vi "photometric acquisitions.vi"(8 "error in (no error)":errorcluster, 11 "S4GEI in":refnum<class "S4GEI.lvclass">) -> (0 "error out":errorcluster, 3 "S4GEI out":refnum<class "S4GEI.lvclass">)   [LabVIEW 2018, in "S4GEI.lvclass"]
uses:
  S4GEI.lvclass
  S4GEI.lvclass/S4GEI.ctl
  State Machine/State Machine.lvclass
  Channel GUI/Channel.lvclass
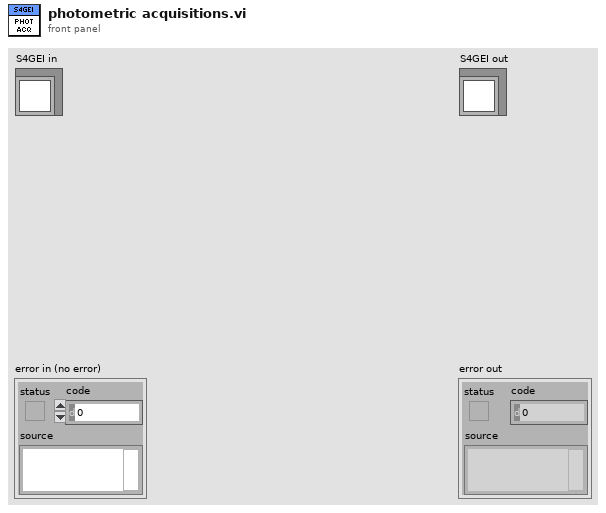
[diagram p1: front panel]
types:
  T1 = cluster{"Acquire":bool, "Stop Acquisition":bool, "Abort Acquisition":bool, "Pause acquisition":bool}
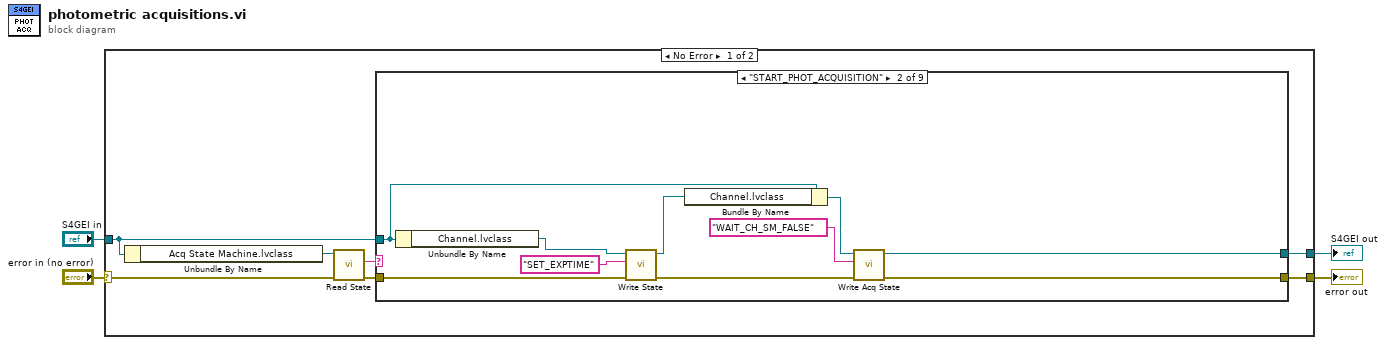
[diagram p0: block diagram]
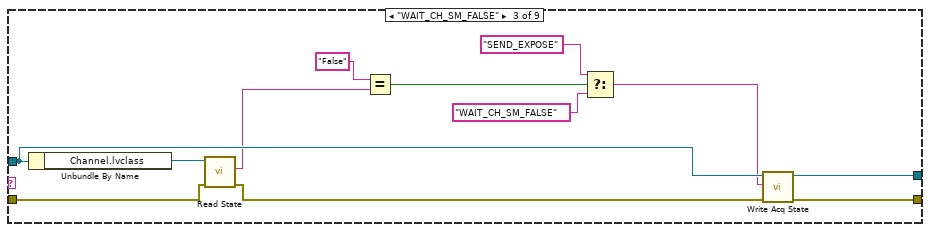
[diagram p3: hidden frame]
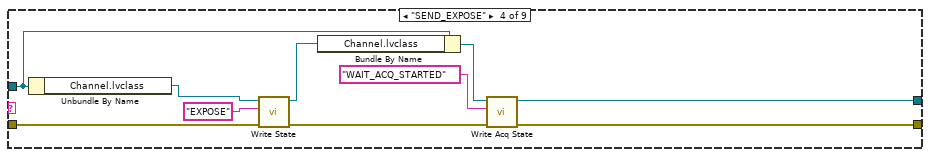
[diagram p4: hidden frame]
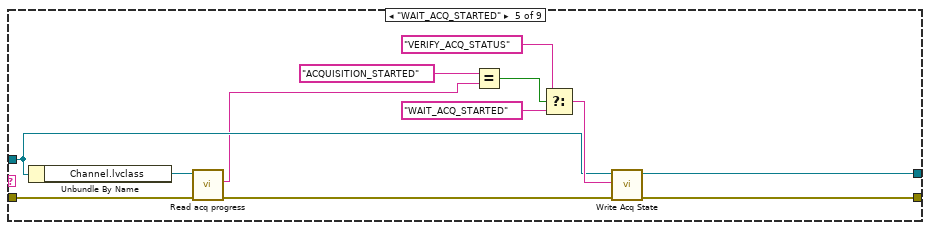
[diagram p5: hidden frame]
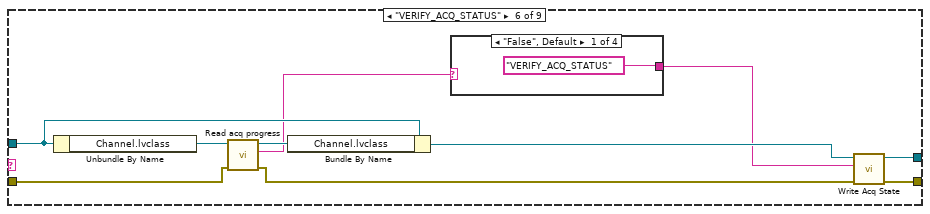
[diagram p6: hidden frame]
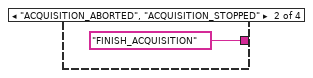
[diagram p7: hidden frame]
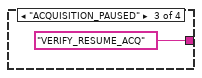
[diagram p8: hidden frame]
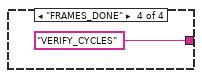
[diagram p9: hidden frame]
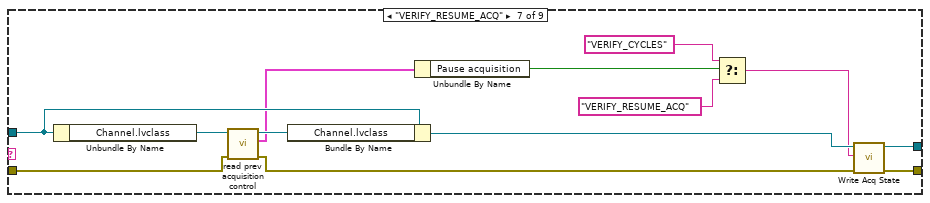
[diagram p10: hidden frame]
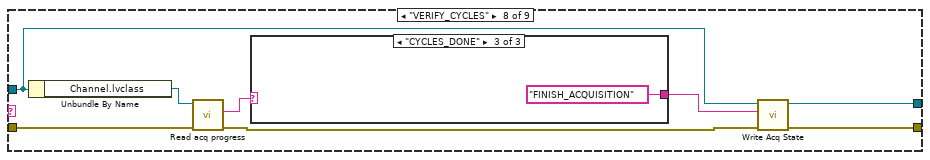
[diagram p11: hidden frame]
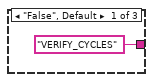
[diagram p12: hidden frame]
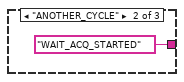
[diagram p13: hidden frame]
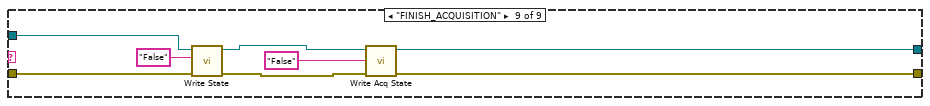
[diagram p14: hidden frame]
diagram:
  n1 = case shown="No Error" "error in (no error)" {
    selector: "error in (no error)" -> [w8 w105]
    tunnel: [w7 w105] -> w3
    tunnel: [w5 w104] -> w1
    tunnel: "S4GEI in" -> [w6 w104]
    frame No Error {
      n2 = Unbundle By Name(w6) -> ("Acq State Machine.lvclass"=w11:refnum<class "State Machine.lvclass">)
      n3 = call-dynamic "Read State.vi"("error in (no error)"=w8, "State Machine in"=w11) -> ("error out"=w9:errorcluster, "State"=w10:string)  [unwired: 7 in, 1 out]
      n4 = case shown="\"START_PHOT_ACQUISITION\"" w10 {
        tunnel: w9 -> [w12 w19 w32 w41 w50 w62 w76 w88 w99]
        tunnel: w6 -> [w13 w16 w31 w38 w52 w67 w82 w90 w100]
        tunnel: [w13 w23 w35 w45 w57 w65 w80 w92 w103] -> w5
        tunnel: [w12 w22 w34 w44 w56 w64 w79 w91 w102] -> w7
        frame "False", Default {
        }
        frame "START_PHOT_ACQUISITION" {
          n5 = Unbundle By Name(w16) -> ("Channel.lvclass"=w20:refnum<class "Channel.lvclass">)
          n6 = call "Write State.vi"("error in (no error)"=w19, "State"="SET_EXPTIME", "Channel GEI in"=w20) -> ("error out"=w17:errorcluster, "Channel GEI out"=w14:refnum<class "Channel.lvclass">)  [unwired: 7 in]
          n7 = Bundle By Name(cluster=w16, "Channel.lvclass"=w14) -> (w15:refnum<class "S4GEI.lvclass">)
          n8 = call "Write Acq State.vi"("error in (no error)"=w17, "State"="WAIT_CH_SM_FALSE" ("x"), "SPARC4_GEI in"=w15) -> ("error out"=w22:errorcluster, "SPARC4_GEI out"=w23:refnum<class "S4GEI.lvclass">)  [unwired: 7 in]
        }
        frame "WAIT_CH_SM_FALSE" {
          n9 = Unbundle By Name(w31) -> ("Channel.lvclass"=w33:refnum<class "Channel.lvclass">)
          n10 = call "Read State.vi"("error in (no error)"=w32, "Channel GEI in"=w33) -> ("error out"=w30:errorcluster, "State"=w29:string)  [unwired: 7 in, 1 out]
          n11 = Equal?(x="False", y=w29) -> (x = y?=w27:bool)
          n12 = Select(t="SEND_EXPOSE" ("x"), s=w27, f="WAIT_CH_SM_FALSE" ("x")) -> (s? t:f=w24:string)
          n13 = call "Write Acq State.vi"("error in (no error)"=w30, "State"=w24, "SPARC4_GEI in"=w31) -> ("error out"=w34:errorcluster, "SPARC4_GEI out"=w35:refnum<class "S4GEI.lvclass">)  [unwired: 7 in]
        }
        frame "SEND_EXPOSE" {
          n14 = Unbundle By Name(w38) -> ("Channel.lvclass"=w42:refnum<class "Channel.lvclass">)
          n15 = call "Write State.vi"("error in (no error)"=w41, "State"="EXPOSE", "Channel GEI in"=w42) -> ("error out"=w39:errorcluster, "Channel GEI out"=w36:refnum<class "Channel.lvclass">)  [unwired: 7 in]
          n16 = Bundle By Name(cluster=w38, "Channel.lvclass"=w36) -> (w37:refnum<class "S4GEI.lvclass">)
          n17 = call "Write Acq State.vi"("error in (no error)"=w39, "State"="WAIT_ACQ_STARTED" ("x"), "SPARC4_GEI in"=w37) -> ("error out"=w44:errorcluster, "SPARC4_GEI out"=w45:refnum<class "S4GEI.lvclass">)  [unwired: 7 in]
        }
        frame "WAIT_ACQ_STARTED" {
          n18 = Unbundle By Name(w52) -> ("Channel.lvclass"=w51:refnum<class "Channel.lvclass">)
          n19 = call-dynamic "Read acq progress.vi"("error in (no error)"=w50, "Channel in"=w51) -> ("error out"=w49:errorcluster, "acq progress"=w48:string)  [unwired: 7 in, 1 out]
          n20 = Equal?(x="ACQUISITION_STARTED" ("State"), y=w48) -> (x = y?=w46:bool)
          n21 = Select(t="VERIFY_ACQ_STATUS" ("State"), s=w46, f="WAIT_ACQ_STARTED" ("State")) -> (s? t:f=w55:string)
          n22 = call "Write Acq State.vi"("error in (no error)"=w49, "State"=w55, "SPARC4_GEI in"=w52) -> ("error out"=w56:errorcluster, "SPARC4_GEI out"=w57:refnum<class "S4GEI.lvclass">)  [unwired: 7 in]
        }
        frame "VERIFY_ACQ_STATUS" {
          n23 = Unbundle By Name(w67) -> ("Channel.lvclass"=w63:refnum<class "Channel.lvclass">)
          n24 = call-dynamic "Read acq progress.vi"("error in (no error)"=w62, "Channel in"=w63) -> ("error out"=w60:errorcluster, "acq progress"=w59:string, "Channel out"=w61:refnum<class "Channel.lvclass">)  [unwired: 7 in]
          n25 = Bundle By Name(cluster=w67, "Channel.lvclass"=w61) -> (w66:refnum<class "S4GEI.lvclass">)
          n26 = case shown="\"False\", Default" w59 {
            tunnel: ["VERIFY_ACQ_STATUS" "FINISH_ACQUISITION" "VERIFY_RESUME_ACQ" "VERIFY_CYCLES"] -> w58
            frame "False", Default {
            }
            frame "ACQUISITION_ABORTED", "ACQUISITION_STOPPED" {
            }
            frame "ACQUISITION_PAUSED" {
            }
            frame "FRAMES_DONE" {
            }
          }
          n27 = call "Write Acq State.vi"("error in (no error)"=w60, "State"=w58, "SPARC4_GEI in"=w66) -> ("error out"=w64:errorcluster, "SPARC4_GEI out"=w65:refnum<class "S4GEI.lvclass">)  [unwired: 7 in]
        }
        frame "VERIFY_RESUME_ACQ" {
          n28 = Unbundle By Name(w82) -> ("Channel.lvclass"=w77:refnum<class "Channel.lvclass">)
          n29 = call-dynamic "read prev acquisition control.vi"("error in (no error)"=w76, "Channel in"=w77) -> ("error out"=w74:errorcluster, "prev acquisition control"=w73:T1, "Channel out"=w75:refnum<class "Channel.lvclass">)  [unwired: 7 in]
          n30 = Bundle By Name(cluster=w82, "Channel.lvclass"=w75) -> (w81:refnum<class "S4GEI.lvclass">)
          n31 = Unbundle By Name(w73) -> ("Pause acquisition"=w72:bool)
          n32 = Select(t="VERIFY_CYCLES", s=w72, f="VERIFY_RESUME_ACQ") -> (s? t:f=w78:string)
          n33 = call "Write Acq State.vi"("error in (no error)"=w74, "State"=w78, "SPARC4_GEI in"=w81) -> ("error out"=w79:errorcluster, "SPARC4_GEI out"=w80:refnum<class "S4GEI.lvclass">)  [unwired: 7 in]
        }
        frame "VERIFY_CYCLES" {
          n34 = Unbundle By Name(w90) -> ("Channel.lvclass"=w89:refnum<class "Channel.lvclass">)
          n35 = call-dynamic "Read acq progress.vi"("error in (no error)"=w88, "Channel in"=w89) -> ("error out"=w87:errorcluster, "acq progress"=w86:string)  [unwired: 7 in, 1 out]
          n36 = case shown="\"CYCLES_DONE\"" w86 {
            tunnel: ["VERIFY_CYCLES" ("State") "WAIT_ACQ_STARTED" ("y") "FINISH_ACQUISITION" ("State")] -> w85
            frame "False", Default {
            }
            frame "ANOTHER_CYCLE" {
            }
            frame "CYCLES_DONE" {
            }
          }
          n37 = call "Write Acq State.vi"("error in (no error)"=w87, "State"=w85, "SPARC4_GEI in"=w90) -> ("error out"=w91:errorcluster, "SPARC4_GEI out"=w92:refnum<class "S4GEI.lvclass">)  [unwired: 7 in]
        }
        frame "FINISH_ACQUISITION" {
          n38 = call "Write State.vi"("error in (no error)"=w99, "State"="False", "SPARC4_GEI in"=w100) -> ("error out"=w98:errorcluster, "SPARC4_GEI out"=w101:refnum<class "S4GEI.lvclass">)  [unwired: 7 in]
          n39 = call "Write Acq State.vi"("error in (no error)"=w98, "State"="False", "SPARC4_GEI in"=w101) -> ("error out"=w102:errorcluster, "SPARC4_GEI out"=w103:refnum<class "S4GEI.lvclass">)  [unwired: 7 in]
        }
      }
    }
    frame Error {
    }
  }
  "error out" <- w3
  "S4GEI out" <- w1
